vi "String to constants arrays.vi"(8 "error in (no error)":errorcluster, 11 "Variables":string) -> (0 "error out":errorcluster, 2 "Variable Names":string[](array[string]), 3 "Array of Numbers":dbl[](array[numeric]))   [LabVIEW 2013]
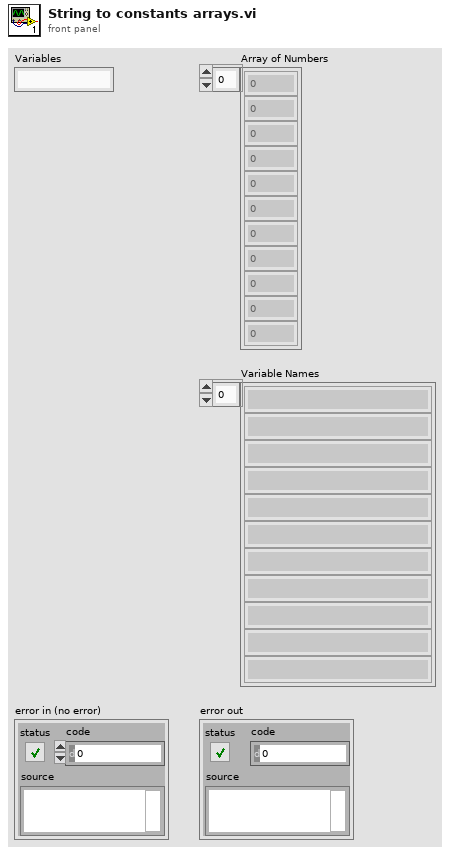
[diagram p1: front panel]
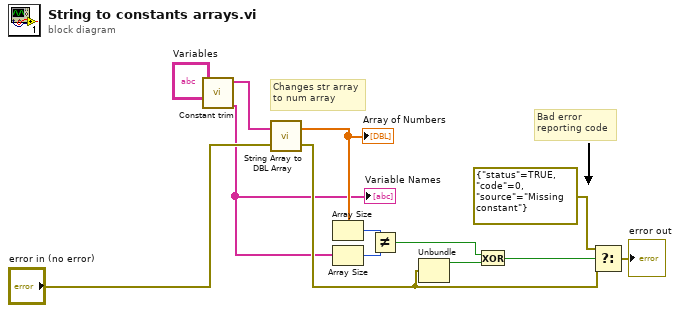
[diagram p0: block diagram]
diagram:
  # "Bad error \nreporting code"
  # "Changes str array\nto num array"
  n1 = call "Constant trim.vi"("String"="Variables") -> ("Array of Names"=w1:string[], "Array of Numbers"=w6:string[])  [unwired: 9 in]
  "Variable Names" <- w1
  n2 = call "String Array to DBL Array.vi"("error in"="error in (no error)", "Array of Numbers"=w6) -> ("Error out"=w9:errorcluster, "Array of Numbers"=w7:dbl[])
  "Array of Numbers" <- w7
  n3 = Array Size(array=w7) -> (size(s)=w3:i32)
  n4 = Array Size(array=w1) -> (size(s)=w2:i32)
  n5 = Not Equal?(x=w3, y=w2) -> (x != y?=w10:bool)
  n6 = Unbundle(w9) -> ("status"=w12:bool)  [unwired: 2 out]
  n7 = Exclusive Or(1:w12, 2:w10) -> (0:w11:bool)
  n8 = Select(t=errorcluster {"status"=TRUE, "code"=0, "source"="Missing constant"} ("error in"), s=w11, f=w9) -> (s? t:f=→"error out":errorcluster)
